vi "Add.vi"(8 "Error In":errorcluster, 10 "IObserver":refnum<class "IObserver.lvclass">, 11 "reference in":refnum<class "CommunicationModule.lvclass">) -> (0 "Error Out":errorcluster, 3 "reference out":refnum<class "CommunicationModule.lvclass">)   [LabVIEW 2024, in "CommunicationModule.lvclass"]
doc: "Add new observer to ObserverList"
uses:
  CommunicationModule.lvclass
  CommunicationModule.lvclass/CommunicationModule.ctl
  IObserver/IObserver.lvclass
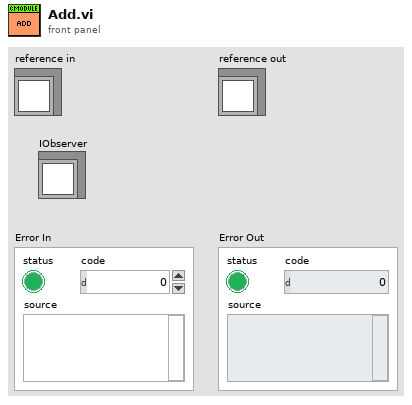
[diagram p1: front panel]
types:
  T1 = typedef "CommunicationModule.lvclass/ObjectAttributes.ctl" = cluster{"ObserverList":refnum<class "IObserver.lvclass">[]}
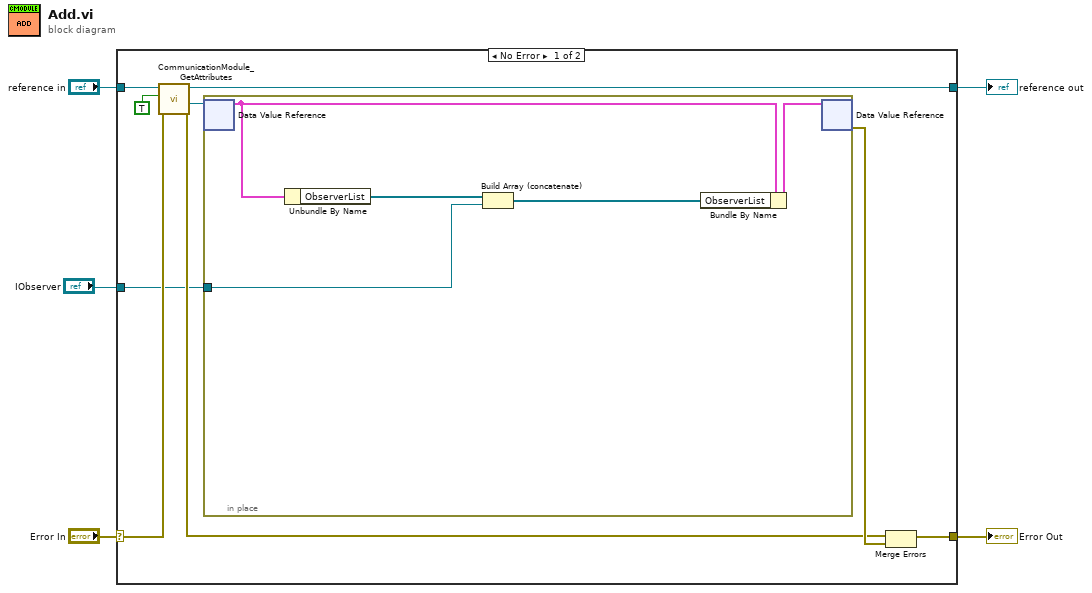
[diagram p0: block diagram]
diagram:
  n1 = case shown="No Error" "Error In" {
    selector: "Error In" -> [w13 w21]
    tunnel: [w10 w21] -> w4
    tunnel: [w11 w20] -> w2
    tunnel: "reference in" -> [w14 w20]
    tunnel: "IObserver" -> [w6 _]
    frame No Error {
      n2 = call "CommunicationModule_GetAttributes.vi"("Error In"=w13, "OnlyGetDvrReference(False)"=TRUE, "reference in"=w14) -> ("Error Out"=w8:errorcluster, "DataRef"=w9:refnum<data-value>, "reference out"=w11:refnum<class "CommunicationModule.lvclass">)  [unwired: 5 in, 1 out]
      n3 = in-place {
        in-place-border: w6 -> [w15]
        n4 = in-place-dvr #1(w9) -> (w18:T1)  [unwired: 1 out]
        n5 = Unbundle By Name(w18) -> ("ObserverList"=w17:refnum<class "IObserver.lvclass">[])
        n6 = Build Array (concatenate)(w17, w15) -> (w16:refnum<class "IObserver.lvclass">[])
        n7 = Bundle By Name(cluster=w18, "ObserverList"=w16) -> (w19:T1)
        n8 = in-place-dvr #1(w19) -> (w12:errorcluster)  [unwired: 1 out]
      }
      n9 = Merge Errors(w8, w12) -> (w10:errorcluster)
    }
    frame Error {
    }
  }
  "Error Out" <- w4
  "reference out" <- w2
